vi "CheckLicens.vi"(8 "error in (no error)":errorcluster) -> (0 "error out":errorcluster, 3 "Dicom Active":bool)   [LabVIEW 2013, in "main.lvlib"]
uses:
  main.lvlib
  Controls/Enum Save Action Events.ctl
  Controls/Enum Variables.ctl
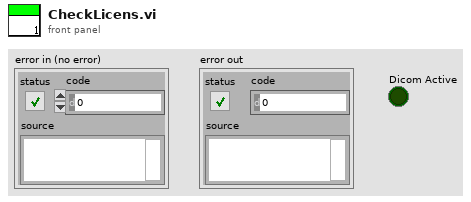
[diagram p1: front panel]
types:
  T1 = typedef "main.lvlib/Enum Variables.ctl" = enum16{"SetAcqFilter", "GetAcqFilter", "Set Filter", "Get Filter", "Set Height", "Get Height", "Set Recorded Height", "Get Recorded Height", "Set Blue Pressure", "Get Blue Pressure", "Set Red Pressure", "Get Red Pressure", "Init", "Reset Pressure", "Set Red Cursors", "Get Red Cursors", "Set Blue Cursors", "Get Blue Cursors", "Set Language", "Get Language", "Set Active Graphs", "Get ActiveGraphs", "Set Method", "Get Method", "Set Encryption", "Get Encryption", "Set ExcelVersion", "Get ExcelVersion", "Set DICOM Avail", "Get DICOM Avail", "Set DICOM Encode", "Get DICOM Encode", "Set JournalExport", "Get JournalExport", "Set Sequence", "Get Sequence", "Set DAQ Connected", "Get DAQ Connected", "Set Current Graph", "Get Current Graph", "Set General Settings", "Get Hyphenation", "Set Arm Calc Method", "Get Arm Calc Method", "Set Dicom Tags", "Get Dicom Tags", "Set BT Serial", "Get BT Serial", "Set BT Accepted Serials", "Get BT Accepted Serials", "Get BT License", "Set BT License"}
  T2 = cluster{"Name":string, "Address":string, "Department":string}
  T3 = typedef "main.lvlib/Enum Save Action Events.ctl" = enum16{"LoadReportPath", "SaveReportPath", "Load Graph Path", "Save Graph Path", "LoadDataPath", "SaveDataPath", "Load Template Path", "Save Template Path", "Load PressureFactor", "Save PressureFactor", "Init", "Load Listbox", "Save Listbox", "LoadHospInfo", "SaveHospInfo", "Load DICOM Activation", "Save DICOM Activation", "LoadDICOMInfoWL", "SaveDICOMInfoWL", "LoadDICOMInfoPACS", "SaveDICOMInfoPACS", "Load ArmCalcMethod", "Save ArmCalcMethod", "LoadItemTags", "SaveItemTags", "LoadDICOMEncoding", "SaveDICOMEncoding", "LoadJournalType", "SaveJournalType", "LoadAcqFilterType", "SaveAcqFilterType", "Load Sequence", "Save Sequence", "Load Acquisition Mode", "Save Acquisition Mode", "Load General Settings", "Save General Settings", "Load Language", "Save Language", "Load Dicom Tags", "Save Dicom Tags", "Load BT Serial", "Save BT Serial", "Load BT License", "Save BT License"}
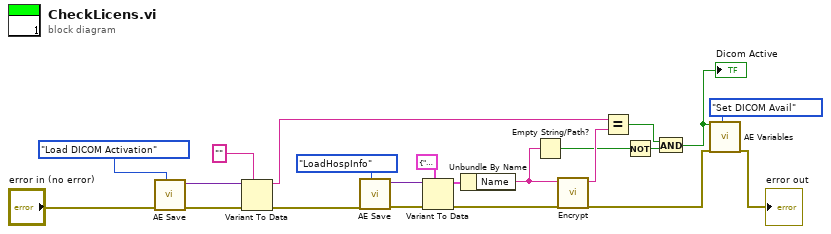
[diagram p0: block diagram]
diagram:
  n1 = call "AE Save.vi"("error in (no error)"="error in (no error)", "Action"=Enum_Save_Action_Events."Load DICOM Activation") -> ("error out"=w14:errorcluster, "Anything"=w12:variant)  [unwired: 7 in]
  n2 = Variant To Data(error in=w14, type="", Variant=w12) -> (data=w10:string, error out=w13:errorcluster)
  n3 = call "AE Save.vi"("error in (no error)"=w13, "Action"=Enum_Save_Action_Events."LoadHospInfo") -> ("error out"=w17:errorcluster, "Anything"=w21:variant)  [unwired: 7 in]
  n4 = Variant To Data(error in=w17, type=T2 {"Name"="", "Address"="", "Department"=""} ("HospInfo"), Variant=w21) -> (data=w15:T2, error out=w8:errorcluster)
  n5 = Unbundle By Name(w15) -> ("Name"=w9:string)
  n6 = Empty String/Path?(string/path=w9) -> (empty?=w3:bool)
  n7 = call "Encrypt.vi"("Input"=w9) -> ("Output"=w5:string)  [unwired: 10 in]
  n8 = Equal?(x=w10, y=w5) -> (x = y?=w2:bool)
  n9 = Not(x=w3) -> (.not. x?=w4:bool)
  n10 = And(x=w2, y=w4) -> (x .and. y?=w1:bool)
  "Dicom Active" <- w1
  n11 = call "AE Variables.vi"("VariantIn"=w1, "error in (no error)"=w8, "Action"=Enum_Variables."Set DICOM Avail") -> ("error out"=→"error out":errorcluster)  [unwired: 9 in, 7 out]
